vi "Add Variable.vi"(8 "error in (no error)":errorcluster, 9 "Variable Name":string, 10 "Variable Type":enum16{"Project", "Execution"}(ring), 11 "Project in":refnum<class "Project.lvclass">) -> (0 "error out":errorcluster, 2 "Variable":cluster{"Name":string, "Value":variant}, 3 "Project out":refnum<class "Project.lvclass">)   [LabVIEW 2015, in "Project.lvclass"]
uses:
  Project.lvclass
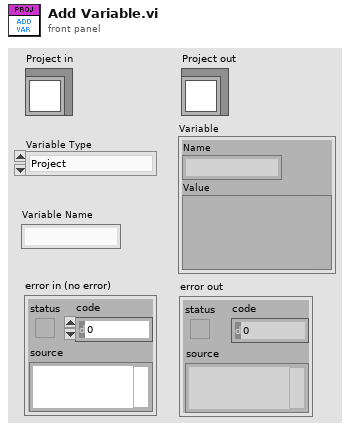
[diagram p1: front panel]
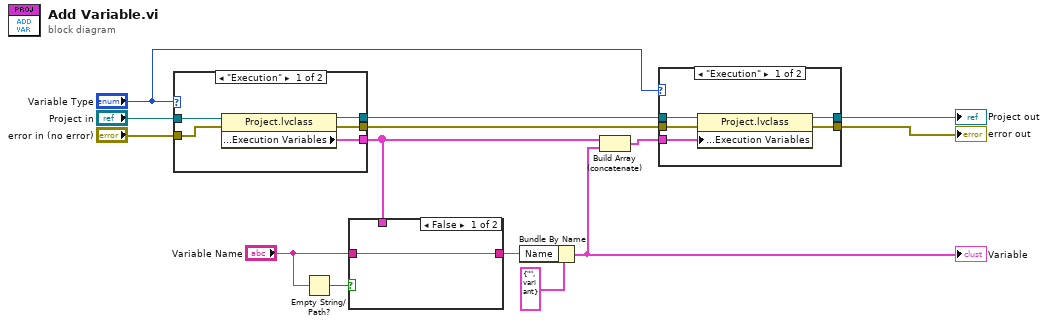
[diagram p0: block diagram]
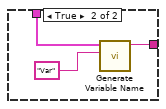
[diagram p2: hidden frame]
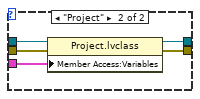
[diagram p3: hidden frame]
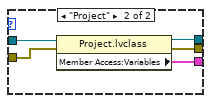
[diagram p4: hidden frame]
diagram:
  n1 = case shown="\"Execution\"" "Variable Type" {
    tunnel: "Project in" -> [w19 w24]
    tunnel: "error in (no error)" -> [w18 w23]
    tunnel: [w17 w22] -> w8
    tunnel: [w16 w21] -> w6
    tunnel: [w15 w20] -> w5
    frame "Execution" {
      n2 = property class="Project.lvclass"(reference=w19, error in=w18) -> (reference out=w16:refnum<class "Project.lvclass">, error out=w15:errorcluster, "Member Access:Execution Variables"=w17:cluster{"Name":string, "Value":variant}[])
    }
    frame "Project" {
      n3 = property class="Project.lvclass"(reference=w24, error in=w23) -> (reference out=w21:refnum<class "Project.lvclass">, error out=w20:errorcluster, "Member Access:Variables"=w22:cluster{"Name":string, "Value":variant}[])
    }
  }
  n4 = Empty String/Path?(string/path="Variable Name") -> (empty?=w2:bool)
  n5 = case shown="False" w2 {
    tunnel: w8 -> [_ w27]
    tunnel: [w25 w26] -> w7
    tunnel: "Variable Name" -> [w25 _]
    frame False {
    }
    frame True {
      n6 = call "Generate Variable Name.vi"("Default Name"="Var", "Variables"=w27) -> ("Name"=w26:string)  [unwired: 9 in]
    }
  }
  n7 = Bundle By Name(cluster=cluster{"Name":string, "Value":variant} {"Name"="", "Value"=variant} ("Variable"), "Name"=w7) -> (w9:cluster{"Name":string, "Value":variant})
  "Variable" <- w9
  n8 = Build Array (concatenate)(w8, w9) -> (w4:cluster{"Name":string, "Value":variant}[])
  n9 = case shown="\"Execution\"" "Variable Type" {
    tunnel: [w33 w38] -> w11
    tunnel: [w32 w37] -> w10
    tunnel: w6 -> [w31 w36]
    tunnel: w5 -> [w30 w35]
    tunnel: w4 -> [w29 w34]
    frame "Execution" {
      n10 = property class="Project.lvclass"(reference=w31, error in=w30, "Member Access:Execution Variables"=w29) -> (reference out=w33:refnum<class "Project.lvclass">, error out=w32:errorcluster)
    }
    frame "Project" {
      n11 = property class="Project.lvclass"(reference=w36, error in=w35, "Member Access:Variables"=w34) -> (reference out=w38:refnum<class "Project.lvclass">, error out=w37:errorcluster)
    }
  }
  "error out" <- w10
  "Project out" <- w11
